vi "Config File UE to CPE.vi"() -> ()   [LabVIEW 2016]
uses:
  <vilib>/Utility/file.llb/Read Delimited Spreadsheet (string).vi
  <vilib>/Utility/file.llb/Write Delimited Spreadsheet (string).vi
panel:
  out "error out":errorcluster
  out "appended array":string[][](array[string])
  in  "file path (dialog if empty)":path
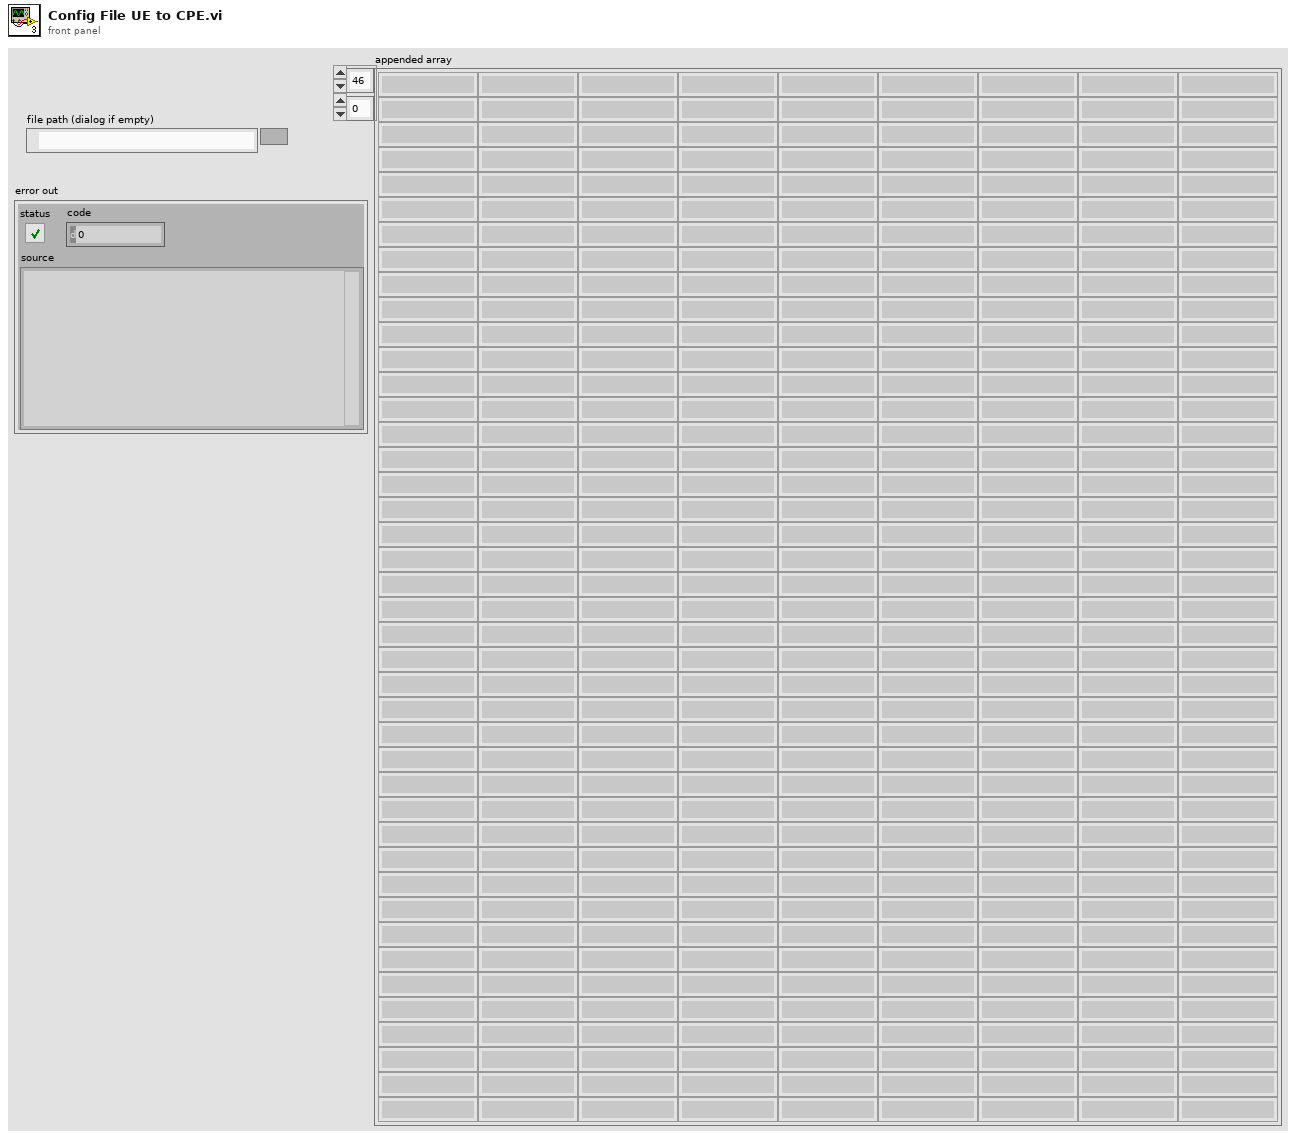
[diagram p1: front panel]
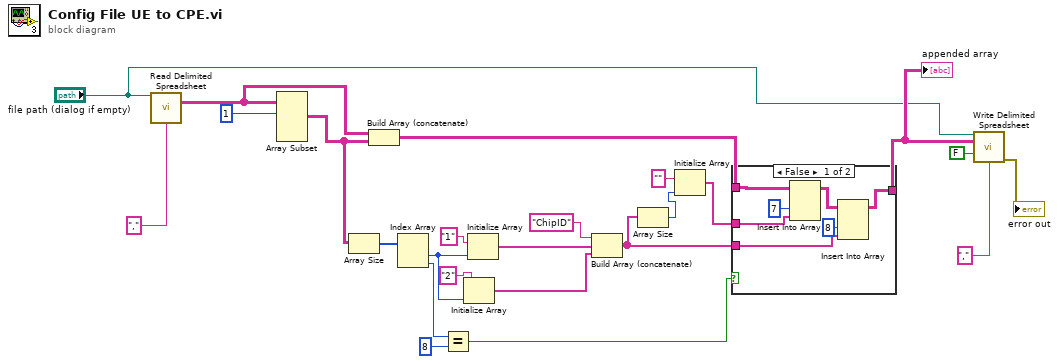
[diagram p0: block diagram]
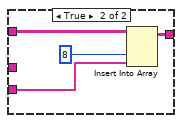
[diagram p2: hidden frame]
diagram:
  n1 = call-poly <vilib>:"Read Delimited Spreadsheet.vi"("file path (dialog if empty)"="file path (dialog if empty)", "delimiter (\\t)"="," ("delimiter (\\t)")) -> ("all rows"=w22:string[][])  [unwired: 8 in, 5 out]
  n2 = Array Subset(array=w22, index (row)=1 ("index")) -> (w20:string[][])  [unwired: 3 in]
  n3 = Array Size(array=w20) -> (size(s)=w19:i32[])
  n4 = Build Array (concatenate)(w22, w20) -> (w21:string[][])
  n5 = Index Array(array=w19) -> (element #1=w17:i32, element #2=w7:i32)  [unwired: 2 in]
  n6 = Equal?(x=w7, y=8) -> (x = y?=w5:bool)
  n7 = Initialize Array("2", w17) -> (w13:string[])
  n8 = Initialize Array("1", w17) -> (w14:string[])
  n9 = Build Array (concatenate)("ChipID", w14, w13) -> (w4:string[])
  n10 = Array Size(array=w4) -> (size(s)=w3:i32)
  n11 = Initialize Array("" ("element"), w3) -> (w1:string[])
  n12 = case shown="False" w5 {
    tunnel: w21 -> [w30 w35]
    tunnel: w4 -> [w26 w33]
    tunnel: [w25 w32] -> w12
    tunnel: w1 -> [w29 _]
    frame False {
      n13 = Insert Into Array(array=w30, index (col)=7 ("disabled index (col)"), new element=w29) -> (w28:string[][])  [unwired: 1 in]
      n14 = Insert Into Array(array=w28, index (col)=8 ("disabled index (col)"), new element=w26) -> (w25:string[][])  [unwired: 1 in]
    }
    frame True {
      n15 = Insert Into Array(array=w35, index (col)=8 ("disabled index (col)"), new element=w33) -> (w32:string[][])  [unwired: 1 in]
    }
  }
  "appended array" <- w12
  n16 = call-poly <vilib>:"Write Delimited Spreadsheet.vi"("file path (dialog if empty)"="file path (dialog if empty)", "2D data"=w12, "append to file? (new file:F)"=FALSE, "delimiter (\\t)"="," ("delimiter (\\t)")) -> ("error out"=→"error out":errorcluster)  [unwired: 10 in, 1 out]
